vi "Time string to time stamp.vi"(8 "error in (no error)":errorcluster, 10 "Time String":string, 11 "OLE DB Timestamp in":refnum<class "OLE DB Timestamp.lvclass">) -> (0 "error out":errorcluster, 2 "Time Stamp":timestamp, 3 "OLE DB Timestamp out":refnum<class "OLE DB Timestamp.lvclass">)   [LabVIEW 2020, in "Basic Columns.lvlib" / "OLE DB Timestamp.lvclass"]
uses:
  OLE DB Timestamp.lvclass
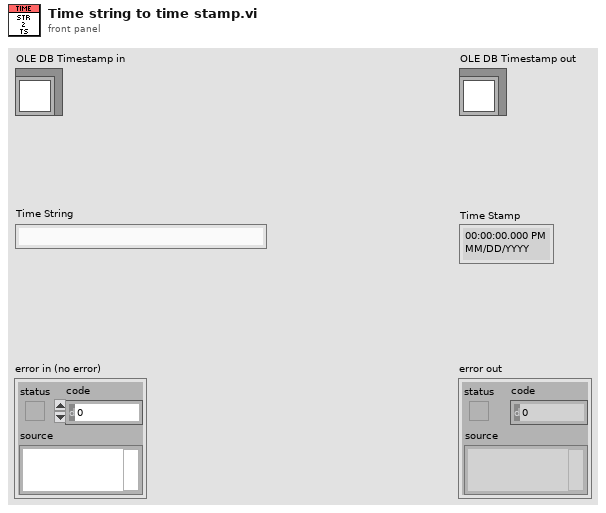
[diagram p1: front panel]
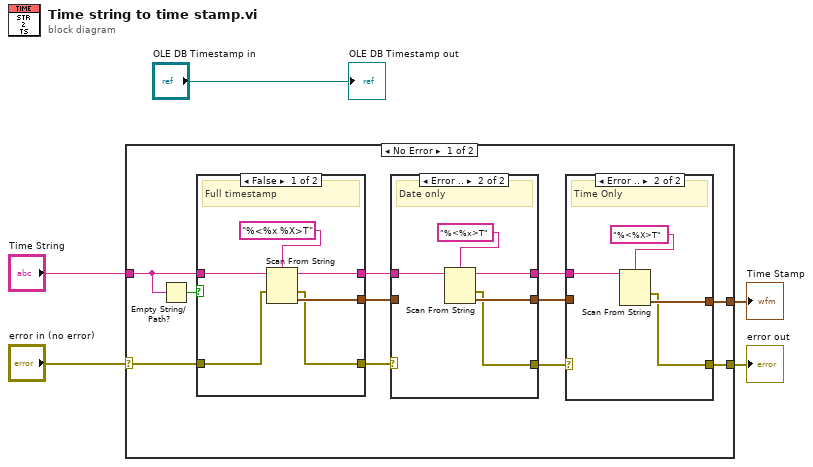
[diagram p0: block diagram]
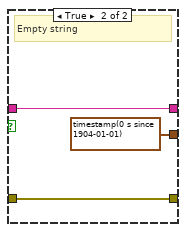
[diagram p4: hidden frame]
diagram:
  n1 = case shown="No Error" "error in (no error)" {
    selector: "error in (no error)" -> [w16 w40]
    tunnel: "Time String" -> [w14 _]
    tunnel: [w7 _] -> w2
    tunnel: [w6 w40] -> w1
    frame No Error {
      n2 = Empty String/Path?(string/path=w14) -> (empty?=w15:bool)
      n3 = case shown="False" w15 {
        tunnel: w14 -> [w35 w37]
        tunnel: [w34 timestamp(0 s since 1904-01-01)] -> w11
        tunnel: w16 -> [w33 w38]
        tunnel: [w32 w38] -> w13
        tunnel: [w31 w37] -> w12
        frame False {
          # "Full timestamp"
          n4 = Scan From String(format string="%<%x %X>T", input string=w35, error in=w33) -> (remaining string=w31:string, error out=w32:errorcluster, output 1=w34:timestamp)  [unwired: 2 in, 1 out]
        }
        frame True {
          # "Empty string"
        }
      }
      n5 = case shown="Error .." w13 {
        selector: w13 -> [w25 _]
        tunnel: [w24 w29] -> w9
        tunnel: [w25 w28] -> w10
        tunnel: w12 -> [w23 w27]
        tunnel: w11 -> [w24 _]
        tunnel: [w23 w26] -> w8
        frame No Error {
          # "Already parsed"
        }
        frame Error {
          # "Date only"
          n6 = Scan From String(format string="%<%x>T", input string=w27) -> (remaining string=w26:string, error out=w28:errorcluster, output 1=w29:timestamp)  [unwired: 3 in, 1 out]
        }
      }
      n7 = case shown="Error .." w10 {
        selector: w10 -> [w18 _]
        tunnel: [w17 w21] -> w7
        tunnel: [w18 w20] -> w6
        tunnel: w8 -> [_ w19]
        tunnel: w9 -> [w17 _]
        frame No Error {
          # "Already Parsed"
        }
        frame Error {
          # "Time Only"
          n8 = Scan From String(format string="%<%X>T", input string=w19) -> (error out=w20:errorcluster, output 1=w21:timestamp)  [unwired: 3 in, 2 out]
        }
      }
    }
    frame Error {
    }
  }
  "error out" <- w1
  "Time Stamp" <- w2
  "OLE DB Timestamp out" <- "OLE DB Timestamp in"
